vi "250224_Cluster_MAJ.vi"(8 "error in (no error)":errorcluster, 9 "Nikon status cluster":T2, 10 "Cluster commandes":T1={"Dia lamp"=TRUE, "Dia lamp intensity"=1689.1304347826087, "Objective"=2, "Light path"=2, "Z pos (µm)"=335593, "Filter wheel 2"=2, "Filter wheel 1"=2, "Shutter 2"=TRUE, "Shutter 1"=TRUE} {"Filter wheel 1" items=["1"=1, "2"=2, "3"=3, "4"=4, "5"=5, "6"=6]; "Filter wheel 2" items=["1"=1, "2"=2, "3"=3, "4"=4, "5"=5, "6"=6]; "Z pos (µm)" min=0 max=990000 step=100 scale=0.0..990000.0; "Light path" items=["1- Eyepiece"=1, "2- Right"=2, "3- Left + Eyepiece"=3, "4- Left"=4]; "Objective" items=["1- Target"=1, "2- PLAN APO 100X 1,45 Oil"=2, "3- Empty"=3, "4- Empty"=4, "5- Empty"=5, "6- Empty"=6]; "Dia lamp intensity" scale=0.0..2100.0}, 11 "Cluster commandes":refnum<vi>) -> (0 "error out":errorcluster, 3 "iLIGHTPATH":i32)   [LabVIEW 2014]
doc: "This vi updates the microscope status cluster.\nThe output is the status of the lightpath (to further display green LEDs accordingly"
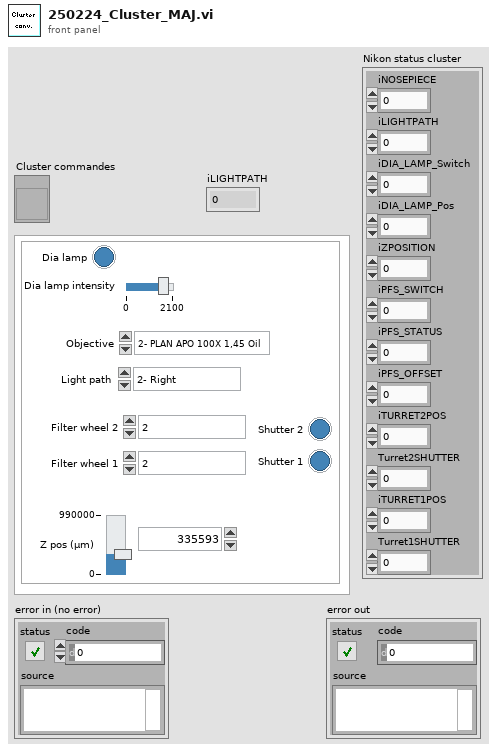
[diagram p1: front panel]
types:
  T1 = cluster{"Dia lamp":bool, "Dia lamp intensity":dbl, "Objective":i32, "Light path":u32, "Z pos (µm)":i32, "Filter wheel 2":u32, "Filter wheel 1":u32, "Shutter 2":bool, "Shutter 1":bool}
  T2 = cluster{"iNOSEPIECE":i32, "iLIGHTPATH":i32, "iDIA_LAMP_Switch":i32, "iDIA_LAMP_Pos":i32, "iZPOSITION":i32, "iPFS_SWITCH":i32, "iPFS_STATUS":i32, "iPFS_OFFSET":i32, "iTURRET2POS":i32, "Turret2SHUTTER":i32, "iTURRET1POS":i32, "Turret1SHUTTER":i32}
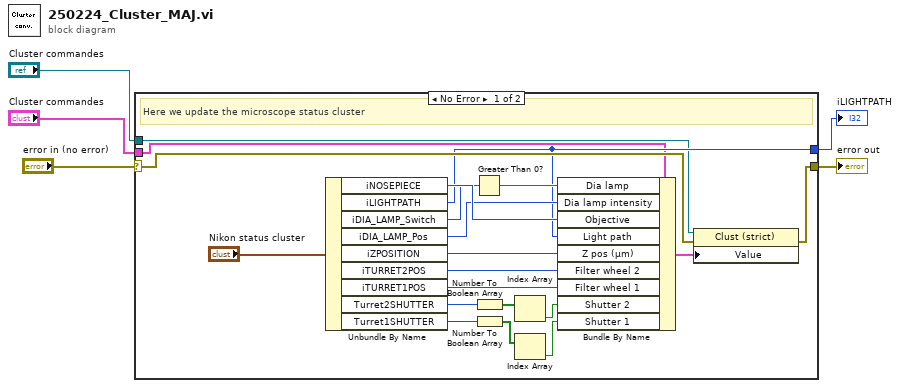
[diagram p0: block diagram]
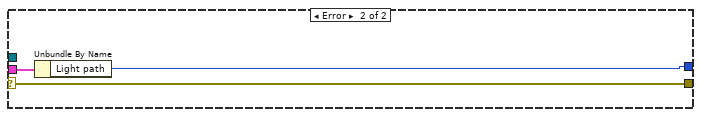
[diagram p2: hidden frame]
diagram:
  n1 = case shown="No Error" "error in (no error)" {
    selector: "error in (no error)" -> [w19 w28]
    tunnel: [w20 w28] -> w5
    tunnel: [w18 w26] -> w3
    tunnel: "Cluster commandes" -> [w17 w27]
    tunnel: "Cluster commandes" -> [w6 _]
    frame No Error {
      # "Here we update the microscope status cluster"
      n2 = Unbundle By Name("Nikon status cluster") -> ("iNOSEPIECE"=w24:i32, "iLIGHTPATH"=w18:i32, "iDIA_LAMP_Switch"=w21:i32, "iDIA_LAMP_Pos"=w22:i32, "iZPOSITION"=w25:i32, "iTURRET2POS"=w14:i32, "iTURRET1POS"=w13:i32, "Turret2SHUTTER"=w12:i32, "Turret1SHUTTER"=w8:i32)
      n3 = Greater Than 0?(x=w21) -> (x > 0?=w23:bool)
      n4 = Number To Boolean Array(number=w12) -> (Boolean array=w11:bool[])
      n5 = Number To Boolean Array(number=w8) -> (Boolean array=w9:bool[])
      n6 = Index Array(array=w11) -> (element=w10:bool)  [unwired: 1 in]
      n7 = Index Array(array=w9) -> (element=w7:bool)  [unwired: 1 in]
      n8 = Bundle By Name(cluster=w17, "Dia lamp"=w23, "Dia lamp intensity"=w22, "Objective"=w24, "Light path"=w18, "Z pos (µm)"=w25, "Filter wheel 2"=w14, "Filter wheel 1"=w13, "Shutter 2"=w10, "Shutter 1"=w7) -> (w16:T1)
      n9 = property on="Property Node" class="Clust (strict)"(reference=w6, error in=w19, "Value"=w16) -> (error out=w20:errorcluster)  [unwired: 1 out]
    }
    frame Error {
      n10 = Unbundle By Name(w27) -> ("Light path"=w26:u32)
    }
  }
  "error out" <- w5
  "iLIGHTPATH" <- w3
